vi "ControlPanel_Basic.vi"() -> ()   [LabVIEW 2009]
uses:
  SubVI's/monochromatorConnect.vi
  SubVI's/monochromatorInitialize.vi
  SubVI's/monochromatorCommandSetWavelength.vi
  SubVI's/monochromatorCommandGetWavelength.vi
  SubVI's/monochromatorCommandSetShutter.vi
  SubVI's/monochromatorCommandGetShutter.vi
  SubVI's/monochromatorDisconnect.vi
  SubVI's/monochromatorCommandSetSteps.vi
panel:
  in  "MainScreenCtrlPanel":enum32{"Page 1"}(tab)
  in  "btn.Shutter":bool
  in  "btn.FastBackward":bool
  in  "btn.Backward":bool
  in  "btn.FastForward":bool
  in  "btn.Forward":bool
  in  "Wavelength":dbl caption="nm" min=0.0 format="%.2f"
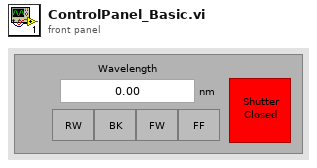
[diagram p1: front panel]
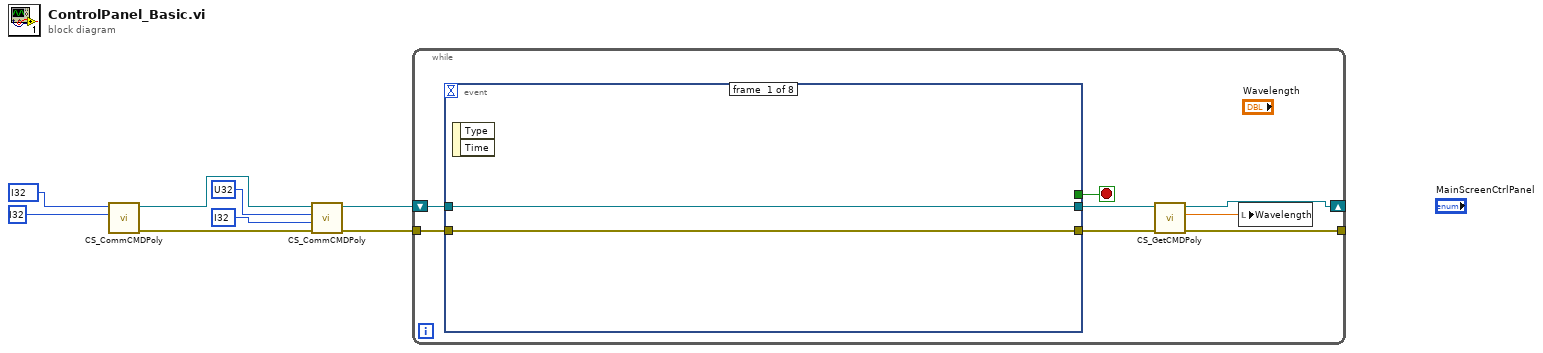
[diagram p0: block diagram]
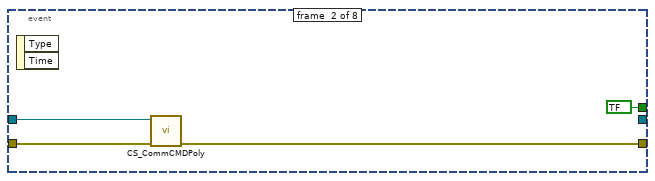
[diagram p2: hidden frame]
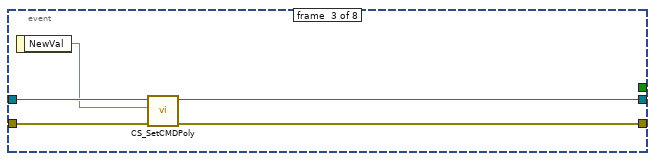
[diagram p3: hidden frame]
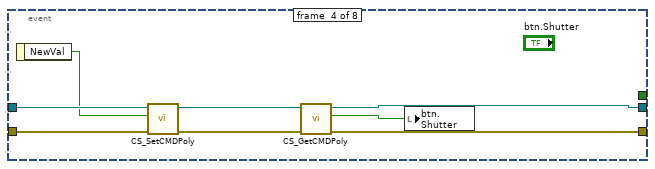
[diagram p4: hidden frame]
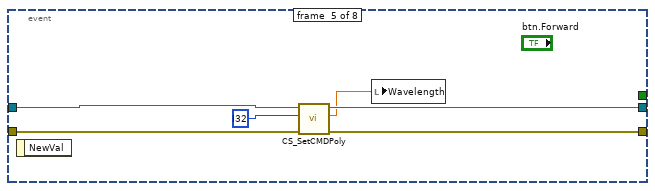
[diagram p5: hidden frame]
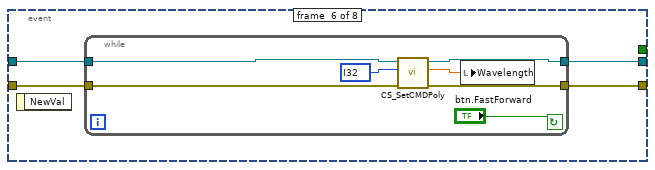
[diagram p6: hidden frame]
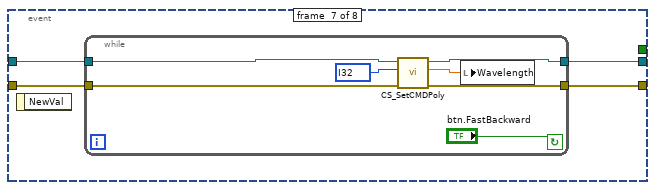
[diagram p7: hidden frame]
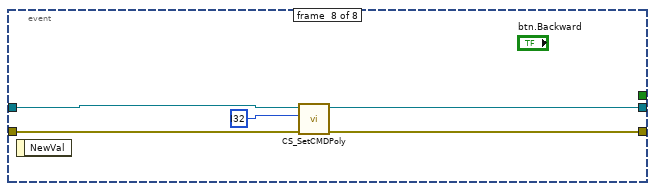
[diagram p8: hidden frame]
diagram:
  n1 = call-poly "CS_CommCMDPoly.vi"("product_id"=i32 ?, "vendor_id"=i32 ?) -> ("error out"=w2:errorcluster, "monochromator"=w8:refnum<k24>)  [unwired: 8 in]
  n2 = call-poly "CS_CommCMDPoly.vi"("error in"=w2, "command_wait_time"=i32 ?, "dev_timeout"=u32 ?, "monochromator"=w8) -> ("error out"=w1:errorcluster, "reference out"=w3:refnum<k24>)  [unwired: 6 in]
  n3 = while {
    tunnel: w1 -> [w14]
    shift-right: [w12] -> _
    shift-left: w3 -> [w15]
    tunnel: [w9] -> _
    stop <- w16 stop-if-true
    n4 = event shown="[5] \"btn.FastForward\": Value Change" {
      selector: _ -> [_ _ _ _ _ _ _ _]
      dyn-events: _ -> [_ _ _ _ _ _ _ _]
      timeout: _ -> [_ _ _ _ _ _ _ _]
      tunnel: [_ bool ? _ _ _ _ _ _] -> w16
      tunnel: w15 -> [w18 w21 w27 w34 w40 w45 w56 w68]
      tunnel: w14 -> [w17 w20 w25 w35 w41 w44 w55 w67]
      tunnel: [w17 w19 w23 w28 w37 w42 w53 w66] -> w10
      tunnel: [w18 _ w24 w31 w38 w43 w54 w65] -> w11
      event #0 {
        n5 = event-data() -> ()  [unwired: 1 in, 2 out]
      }
      event #1 {
        n6 = event-data() -> ()  [unwired: 1 in, 2 out]
        n7 = call-poly "CS_CommCMDPoly.vi"("error in"=w20, "monochromator"=w21) -> ("error out"=w19:errorcluster)  [unwired: 9 in]
      }
      event #2 {
        n8 = event-data() -> ("NewVal"=w26:dbl)  [unwired: 1 in]
        n9 = call-poly "CS_SetCMDPoly.vi"("error in"=w25, "wavelength"=w26, "monochromator"=w27) -> ("error out"=w23:errorcluster, "monochromator"=w24:refnum<k24>)  [unwired: 6 in, 1 out]
      }
      event #3 {
        n10 = event-data() -> ("NewVal"=w33:bool)  [unwired: 1 in]
        n11 = call-poly "CS_SetCMDPoly.vi"("error in"=w35, "shutter"=w33, "monochromator"=w34) -> ("error out"=w29:errorcluster, "monochromator"=w32:refnum<k24>)  [unwired: 7 in]
        n12 = call-poly "CS_GetCMDPoly.vi"("error in"=w29, "monochromator"=w32) -> ("error out"=w28:errorcluster, "shutter"=w30:bool, "monochromator"=w31:refnum<k24>)  [unwired: 6 in, 1 out]
        n13 = local write "btn.Shutter"(w30) -> ()
      }
      event #4 {
        n14 = event-data() -> ()  [unwired: 1 in, 1 out]
        n15 = call-poly "CS_SetCMDPoly.vi"("error in"=w41, "step"=i32 ?, "monochromator"=w40) -> ("error out"=w37:errorcluster, "wavelength"=w36:dbl, "monochromator"=w38:refnum<k24>)  [unwired: 6 in]
        n16 = local write "Wavelength"(w36) -> ()
      }
      event #5 {
        n17 = event-data() -> ()  [unwired: 1 in, 1 out]
        n18 = while {
          tunnel: w45 -> [w52]
          tunnel: w44 -> [w51]
          tunnel: [w46] -> w43
          tunnel: [w47] -> w42
          stop <- "btn.FastForward" continue-if-true
          n19 = call-poly "CS_SetCMDPoly.vi"("error in"=w51, "step"=i32 ?, "monochromator"=w52) -> ("error out"=w47:errorcluster, "wavelength"=w48:dbl, "monochromator"=w46:refnum<k24>)  [unwired: 6 in]
          n20 = local write "Wavelength"(w48) -> ()
        }
      }
      event #6 {
        n21 = event-data() -> ()  [unwired: 1 in, 1 out]
        n22 = while {
          tunnel: [w58] -> w54
          tunnel: [w59] -> w53
          tunnel: w56 -> [w62]
          tunnel: w55 -> [w61]
          stop <- "btn.FastBackward" continue-if-true
          n23 = call-poly "CS_SetCMDPoly.vi"("error in"=w61, "step"=i32 ?, "monochromator"=w62) -> ("error out"=w59:errorcluster, "wavelength"=w57:dbl, "monochromator"=w58:refnum<k24>)  [unwired: 6 in]
          n24 = local write "Wavelength"(w57) -> ()
        }
      }
      event #7 {
        n25 = event-data() -> ()  [unwired: 1 in, 1 out]
        n26 = call-poly "CS_SetCMDPoly.vi"("error in"=w67, "step"=i32 ?, "monochromator"=w68) -> ("error out"=w66:errorcluster, "monochromator"=w65:refnum<k24>)  [unwired: 6 in, 1 out]
      }
    }
    n27 = call-poly "CS_GetCMDPoly.vi"("error in"=w10, "monochromator"=w11) -> ("error out"=w9:errorcluster, "wavelength"=w13:dbl, "monochromator"=w12:refnum<k24>)  [unwired: 7 in]
    n28 = local write "Wavelength"(w13) -> ()
  }
